vi "sendCommand.vi"(6 "Address":i32, 7 "Data":i32, 8 "error in":errorcluster, 9 "Action":u16(ring)=1 items=["sendCommand"=9, "FPGA_writeRegister"=3, "FPGA_readRegister"=2, "uC_writeRegister"=1, "uC_readRegister"=0], 10 "id_in":i32, 11 "connection ID":refnum<k5>) -> (0 "error out":errorcluster, 1 "id_out":i32, 2 "Data out":string, 3 "connection ID out":refnum<k5>, 4 "bytes written":i32)   [LabVIEW 2012]
doc: "This VI sends a command to the Integration Board and provides the received data when necessary."
panel:
  out "String":string
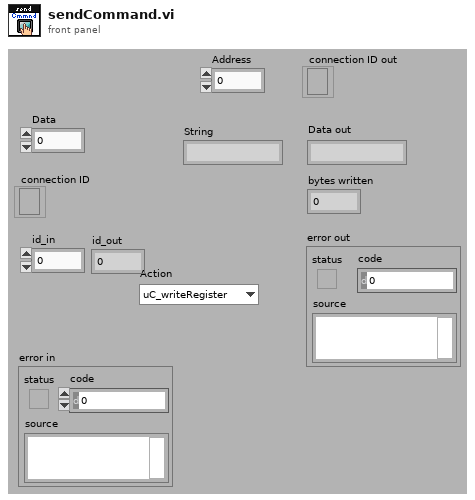
[diagram p1: front panel]
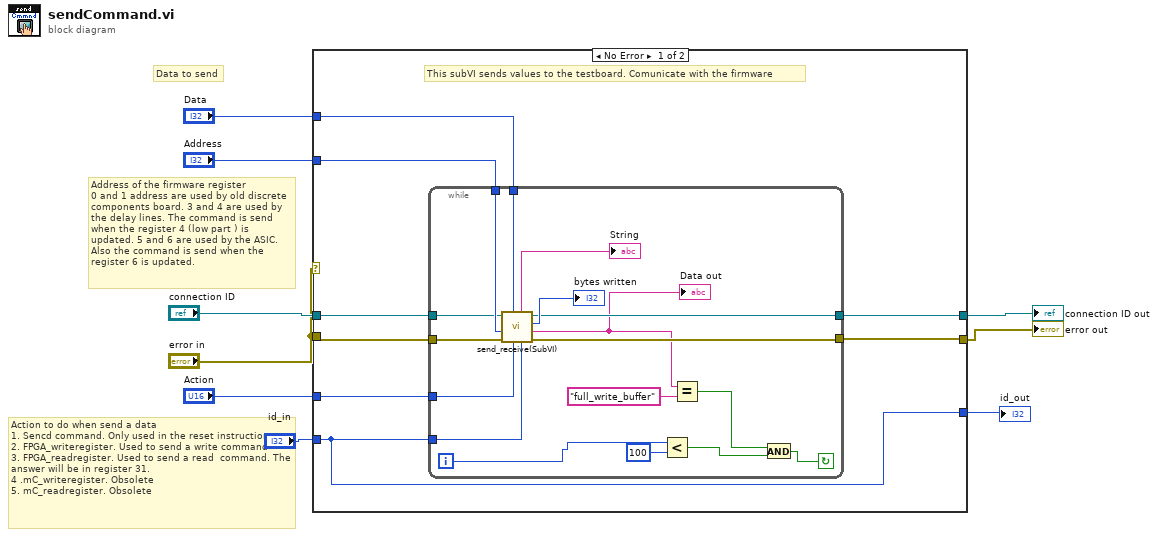
[diagram p0: block diagram]
diagram:
  # "Action to do when send a data\n1. Sencd command. Only used in the reset instruction\n2. FPGA_writeregister. Used to send a write command\n3. FPGA_readregister. Used to send a read  command. The answer will be in register 31.\n4 .mC_writeregister. Obsolete\n5. mC_readregister. Obsolete"
  # "Data to send"
  # "Address of the firmware register\n0 and 1 address are used by old discrete components board. 3 and 4 are used by the delay lines. The command is send when the register 4 (low part ) is updated. 5 and 6 are used by the ASIC. Also the command is send when the register 6 is updated."
  n1 = case shown="No Error" "error in" {
    tunnel: "id_in" -> [w10 w35]
    tunnel: "error in" -> [w13 w36]
    tunnel: "connection ID" -> [w14 w37]
    tunnel: [w11 w36] -> w7
    tunnel: [w12 w37] -> w6
    tunnel: "Data" -> [w17 _]
    tunnel: "Address" -> [w16 _]
    tunnel: "Action" -> [w15 _]
    tunnel: [w10 w35] -> w1
    frame No Error {
      # "This subVI sends values to the testboard. Comunicate with the firmware"
      n2 = while {
        tunnel: w17 -> [w34]
        tunnel: w16 -> [w33]
        tunnel: w15 -> [w32]
        tunnel: w14 -> [w30]
        tunnel: w13 -> [w29]
        tunnel: [w28] -> w12
        tunnel: [w27] -> w11
        tunnel: w10 -> [w25]
        i -> [w19]
        stop <- w22 continue-if-true
        n3 = call "send_receive(SubVI).vi"("id"=w25, "Action"=w32, "Data"=w34, "error in"=w29, "Address"=w33, "connection ID"=w30) -> ("error out"=w27:errorcluster, "data out"=w24:string, "bytes written"=→"bytes written":i32, "connection ID out"=w28:refnum<k5>, "String"=→"String":string)  [unwired: 1 in]
        "Data out" <- w24
        n4 = Less?(x=w19, y=100) -> (x < y?=w20:bool)
        n5 = Equal?(x=w24, y="full_write_buffer") -> (x = y?=w21:bool)
        n6 = And(x=w21, y=w20) -> (x .and. y?=w22:bool)
      }
    }
    frame Error {
    }
  }
  "error out" <- w7
  "connection ID out" <- w6
  "id_out" <- w1
